vi "Method.vi"(4 "Value B":refnum<class "Abs_Numeric.lvclass">, 5 "Value A":refnum<class "Complex Extended Float.lvclass">) -> (1 "Result":refnum<class "Abs_Boolean.lvclass">)   [LabVIEW 2021, in "Less_CPLX_EXT.lvclass"]
uses:
  Less_CPLX_EXT.lvclass
  Less_CPLX_EXT.lvclass/Less_CPLX_EXT.ctl
  Abs_Types/Complex Extended Float/Complex Extended Float.lvclass
  C:/Users/Tim/Documents/GitHub/LV_Abstract/Source/Abs_Types/Floating Point/Abs_Floating Point.lvclass
  C:/Users/Tim/Documents/GitHub/LV_Abstract/Source/Abs_Types/Numeric/Abs_Numeric.lvclass
  C:/Users/Tim/Documents/GitHub/LV_Abstract/Source/Abs_Types/Value/Abs_Value.lvclass
  C:/Users/Tim/Documents/GitHub/LV_Abstract/Source/Abs_Types/Type/Abs_Type.lvclass
  C:/Users/Tim/Documents/GitHub/LV_Abstract/Source/Abs_Types/Complex Extended Float/Complex Extended Float.lvclass
  C:/Users/Tim/Documents/GitHub/LV_Abstract/Source/Functions/Support/Compare/Two Term/CPLX_EXT/AbsComp_Two Term_CPLX_EXT.lvclass
  C:/Users/Tim/Documents/GitHub/LV_Abstract/Source/Abs_Types/Boolean/Abs_Boolean.lvclass
  C:/Users/Tim/Documents/GitHub/LV_Abstract/Source/Functions/Compare/Support/Less/CPLX_EXT/Less_CPLX_EXT.lvclass
  Abs_Types/Boolean/Abs_Boolean.lvclass
  Abs_Types/Numeric/Abs_Numeric.lvclass
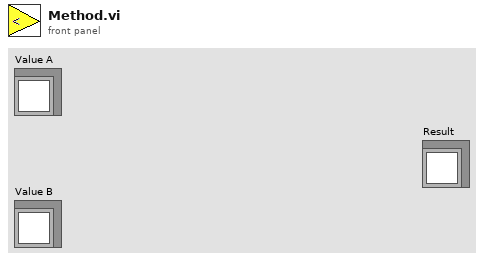
[diagram p1: front panel]
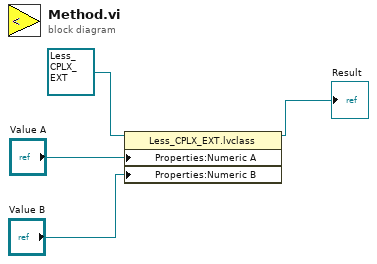
[diagram p0: block diagram]
diagram:
  n1 = property class="Less_CPLX_EXT.lvclass"(reference=refnum<class "Less_CPLX_EXT.lvclass"> refnum ("Greater 0_U64.lvclass"), "Properties:Numeric A"="Value A", "Properties:Numeric B"="Value B") -> (reference out=→"Result":refnum<class "Less_CPLX_EXT.lvclass">)  [unwired: 1 in, 1 out]
